vi "Axis_Initialisation.vi"(4 "Character Size":sgl=0.5, 5 "Half plane?":bool=TRUE, 6 "Axis label?":bool, 7 "Color 2":u32(colorbox)=1244928, 8 "error in (no error)":errorcluster, 9 "Radius":sgl=0.01, 10 "Length":sgl=2.0, 11 "Name":string="XYZ axis") -> (0 "error out":errorcluster, 3 "New Object Refnum":refnum<vi>)   [LabVIEW 2015]
uses:
  <vilib>/Utility/miscctls.llb/LVSceneTextAlignment.ctl
  <vilib>/picture/3D Picture Control/Object/Create Object (name).vi
  <vilib>/picture/3D Picture Control/Object/Create Object (drawable).vi
  <vilib>/picture/3D Picture Control/Object/Add Object (no reference).vi
  <vilib>/picture/3D Picture Control/NI_3D Picture Control.lvlib
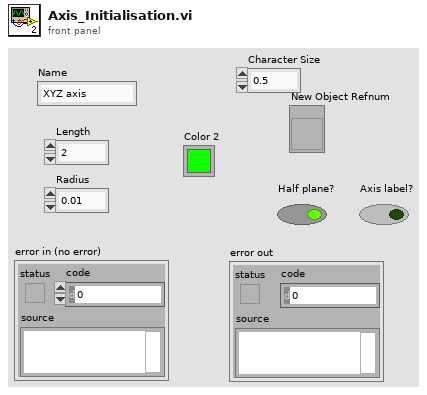
[diagram p1: front panel]
types:
  T1 = typedef "LVSceneTextAlignment.ctl" = cluster{"Horizontal Alignment":enum8{"Left", "Right", "Center"}, "Vertical Alignment":enum8{"Top", "Bottom", "Center", "Base Line", "Bottom Base Line"}}
  T2 = cluster{"Alignment":T1, "Axis Alignment":enum8{"X-Y", "Y-Z", "X-Z", "Reversed X-Y", "Reversed Y-Z", "Reversed X-Z", "Screen"}, "Vertical?":bool, "Wrap Distance":sgl}
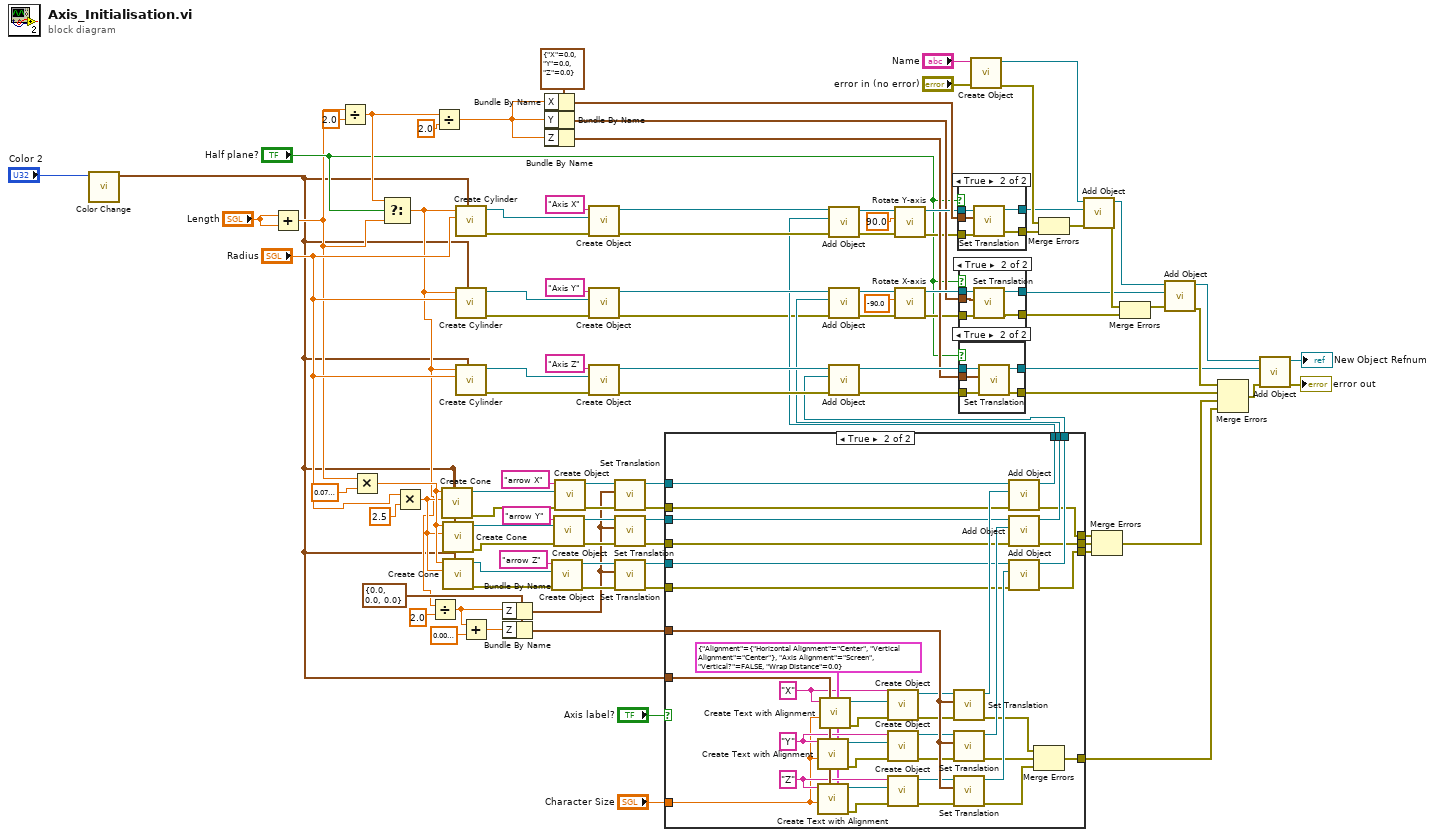
[diagram p0: block diagram]
diagram:
  w51 = cluster{"X":sgl, "Y":sgl, "Z":sgl} {"X"=0.0, "Y"=0.0, "Z"=0.0} ("Translation")
  w36 = cluster{"X":sgl, "Y":sgl, "Z":sgl} {"X"=0.0, "Y"=0.0, "Z"=0.0} ("Translation")
  n1 = call <vilib>:"Color Change.vi"("Color"="Color 2") -> ("RGBA"=w1:cluster{"R":sgl, "G":sgl, "B":sgl, "A":sgl})  [unwired: 10 in]
  n2 = Add(x="Length", y="Length") -> (x+y=w4:sgl)
  n3 = Divide(x=w4, y=sgl 2.0) -> (x/y=w72:sgl)
  n4 = Multiply(x=w4, y=sgl 0.08) -> (x*y=w14:sgl)
  n5 = Select(t=w72, s="Half plane?", f=w4) -> (s? t:f=w3:sgl)
  n6 = Multiply(x="Radius", y=sgl 2.5) -> (x*y=w13:sgl)
  n7 = Divide(x=w3, y=sgl 2.0 ("x")) -> (x/y=w15:sgl)
  n8 = Divide(x=w72, y=sgl 2.0) -> (x/y=w50:sgl)
  n9 = call <vilib>:"Create Cone.vi"("Color"=w1, "Radius"=w13, "Height"=w14) -> ("error out"=w16:errorcluster, "New Cone Refnum"=w58:refnum<vi>)  [unwired: 7 in]
  n10 = call <vilib>:"Create Cone.vi"("Color"=w1, "Radius"=w13, "Height"=w14) -> ("error out"=w9:errorcluster, "New Cone Refnum"=w11:refnum<vi>)  [unwired: 7 in]
  n11 = call <vilib>:"Create Cone.vi"("Color"=w1, "Radius"=w13, "Height"=w14) -> ("error out"=w10:errorcluster, "New Cone Refnum"=w12:refnum<vi>)  [unwired: 7 in]
  n12 = call <vilib>:"Create Cylinder.vi"("Color"=w1, "Radius"="Radius", "Height"=w3) -> ("error out"=w88:errorcluster, "New Cylinder Refnum"=w94:refnum<vi>)  [unwired: 7 in]
  n13 = call <vilib>:"Create Cylinder.vi"("Color"=w1, "Radius"="Radius", "Height"=w3) -> ("error out"=w87:errorcluster, "New Cylinder Refnum"=w96:refnum<vi>)  [unwired: 7 in]
  n14 = call <vilib>:"Create Cylinder.vi"("Color"=w1, "Radius"="Radius", "Height"=w3) -> ("error out"=w86:errorcluster, "New Cylinder Refnum"=w95:refnum<vi>)  [unwired: 7 in]
  n15 = Add(x=w15, y=sgl 0.01) -> (x+y=w27:sgl)
  n16 = Bundle By Name(cluster=w36, "Z"=w15) -> (w47:cluster{"X":sgl, "Y":sgl, "Z":sgl})
  n17 = Bundle By Name(cluster=w36, "Z"=w27) -> (w32:cluster{"X":sgl, "Y":sgl, "Z":sgl})
  n18 = Bundle By Name(cluster=w51, "X"=w50) -> (w74:cluster{"X":sgl, "Y":sgl, "Z":sgl})
  n19 = Bundle By Name(cluster=w51, "Y"=w50) -> (w52:cluster{"X":sgl, "Y":sgl, "Z":sgl})
  n20 = Bundle By Name(cluster=w51, "Z"=w50) -> (w49:cluster{"X":sgl, "Y":sgl, "Z":sgl})
  n21 = call-poly <vilib>:"Create Object.vi"("error in (no error)"=w10, "Geometry"=w12, "Name"="arrow Z") -> ("error out"=w59:errorcluster, "Scene:New Object"=w60:refnum<vi>)  [unwired: 7 in]
  n22 = call-poly <vilib>:"Create Object.vi"("error in (no error)"=w9, "Geometry"=w11, "Name"="arrow Y") -> ("error out"=w64:errorcluster, "Scene:New Object"=w63:refnum<vi>)  [unwired: 7 in]
  n23 = call-poly <vilib>:"Create Object.vi"("error in (no error)"=w16, "Geometry"=w58, "Name"="arrow X") -> ("error out"=w77:errorcluster, "Scene:New Object"=w78:refnum<vi>)  [unwired: 7 in]
  n24 = call-poly <vilib>:"Create Object.vi"("error in (no error)"=w88, "Geometry"=w94, "Name"="Axis X") -> ("error out"=w42:errorcluster, "Scene:New Object"=w67:refnum<vi>)  [unwired: 7 in]
  n25 = call-poly <vilib>:"Create Object.vi"("error in (no error)"=w87, "Geometry"=w96, "Name"="Axis Y") -> ("error out"=w19:errorcluster, "Scene:New Object"=w62:refnum<vi>)  [unwired: 7 in]
  n26 = call-poly <vilib>:"Create Object.vi"("error in (no error)"=w86, "Geometry"=w95, "Name"="Axis Z") -> ("error out"=w46:errorcluster, "Scene:New Object"=w57:refnum<vi>)  [unwired: 7 in]
  n27 = call <vilib>:"Set Translation.vi"("error in (no error)"=w77, "Translation"=w47, "Scene Object"=w78) -> ("error out"=w26:errorcluster, "Translated Object"=w38:refnum<vi>)  [unwired: 7 in]
  n28 = call <vilib>:"Set Translation.vi"("error in (no error)"=w64, "Translation"=w47, "Scene Object"=w63) -> ("error out"=w25:errorcluster, "Translated Object"=w35:refnum<vi>)  [unwired: 7 in]
  n29 = call <vilib>:"Set Translation.vi"("error in (no error)"=w59, "Translation"=w47, "Scene Object"=w60) -> ("error out"=w28:errorcluster, "Translated Object"=w33:refnum<vi>)  [unwired: 7 in]
  n30 = case shown="True" "Axis label?" {
    tunnel: w38 -> [w109 w146]
    tunnel: [w109 w145] -> w37
    tunnel: w35 -> [w108 w144]
    tunnel: [w108 w142] -> w34
    tunnel: w33 -> [w104 w141]
    tunnel: w32 -> [_ w140]
    tunnel: [w104 w138] -> w31
    tunnel: w28 -> [w106 w137]
    tunnel: w26 -> [w107 w136]
    tunnel: w25 -> [w105 w135]
    tunnel: [w107 w134] -> w24
    tunnel: [w105 w133] -> w23
    tunnel: [w106 w132] -> w22
    tunnel: [_ w131] -> w20
    tunnel: w1 -> [_ w130]
    tunnel: "Character Size" -> [_ w110]
    frame False {
    }
    frame True {
      w122 = "Z" ("text")
      w127 = "Y" ("text")
      w117 = T2 {"Alignment"={"Horizontal Alignment"=enum."Center", "Vertical Alignment"=enum."Center"}, "Axis Alignment"=enum."Screen", "Vertical?"=FALSE, "Wrap Distance"=0.0} ("Font options")
      w115 = "X" ("text")
      n31 = call <vilib>:"Create Text with Alignment.vi"("Font Options"=w117, "Color"=w130, "Character Size"=w110, "Text"=w127) -> ("error out"=w119:errorcluster, "New Text Refnum"=w126:refnum<vi>)  [unwired: 6 in]
      n32 = call <vilib>:"Create Text with Alignment.vi"("Font Options"=w117, "Color"=w130, "Character Size"=w110, "Text"=w122) -> ("error out"=w121:errorcluster, "New Text Refnum"=w123:refnum<vi>)  [unwired: 6 in]
      n33 = call <vilib>:"Create Text with Alignment.vi"("Font Options"=w117, "Color"=w130, "Character Size"=w110, "Text"=w115) -> ("error out"=w114:errorcluster, "New Text Refnum"=w129:refnum<vi>)  [unwired: 6 in]
      n34 = call-poly <vilib>:"Create Object.vi"("error in (no error)"=w114, "Geometry"=w129, "Name"=w115) -> ("error out"=w116:errorcluster, "Scene:New Object"=w128:refnum<vi>)  [unwired: 7 in]
      n35 = call-poly <vilib>:"Create Object.vi"("error in (no error)"=w119, "Geometry"=w126, "Name"=w127) -> ("error out"=w118:errorcluster, "Scene:New Object"=w125:refnum<vi>)  [unwired: 7 in]
      n36 = call-poly <vilib>:"Create Object.vi"("error in (no error)"=w121, "Geometry"=w123, "Name"=w122) -> ("error out"=w120:errorcluster, "Scene:New Object"=w124:refnum<vi>)  [unwired: 7 in]
      n37 = call <vilib>:"Set Translation.vi"("error in (no error)"=w116, "Translation"=w140, "Scene Object"=w128) -> ("error out"=w111:errorcluster, "Translated Object"=w147:refnum<vi>)  [unwired: 7 in]
      n38 = call <vilib>:"Set Translation.vi"("error in (no error)"=w118, "Translation"=w140, "Scene Object"=w125) -> ("error out"=w112:errorcluster, "Translated Object"=w143:refnum<vi>)  [unwired: 7 in]
      n39 = call <vilib>:"Set Translation.vi"("error in (no error)"=w120, "Translation"=w140, "Scene Object"=w124) -> ("error out"=w113:errorcluster, "Translated Object"=w139:refnum<vi>)  [unwired: 7 in]
      n40 = call-poly <vilib>:"Add Object.vi"("error in (no error)"=w136, "New Object In"=w147, "Scene Object In"=w146) -> ("error out"=w134:errorcluster, "Scene Object Out"=w145:refnum<vi>)  [unwired: 7 in]
      n41 = call-poly <vilib>:"Add Object.vi"("error in (no error)"=w135, "New Object In"=w143, "Scene Object In"=w144) -> ("error out"=w133:errorcluster, "Scene Object Out"=w142:refnum<vi>)  [unwired: 7 in]
      n42 = call-poly <vilib>:"Add Object.vi"("error in (no error)"=w137, "New Object In"=w139, "Scene Object In"=w141) -> ("error out"=w132:errorcluster, "Scene Object Out"=w138:refnum<vi>)  [unwired: 7 in]
      n43 = Merge Errors(w111, w112, w113) -> (w131:errorcluster)
    }
  }
  n44 = call-poly <vilib>:"Add Object.vi"("error in (no error)"=w42, "New Object In"=w37, "Scene Object In"=w67) -> ("error out"=w41:errorcluster, "Scene Object Out"=w66:refnum<vi>)  [unwired: 7 in]
  n45 = call-poly <vilib>:"Add Object.vi"("error in (no error)"=w19, "New Object In"=w34, "Scene Object In"=w62) -> ("error out"=w18:errorcluster, "Scene Object Out"=w61:refnum<vi>)  [unwired: 7 in]
  n46 = call-poly <vilib>:"Add Object.vi"("error in (no error)"=w46, "New Object In"=w31, "Scene Object In"=w57) -> ("error out"=w45:errorcluster, "Scene Object Out"=w54:refnum<vi>)  [unwired: 7 in]
  n47 = call <vilib>:"Rotate Y-axis.vi"("error in (no error)"=w41, "angle"=90.0, "Scene Object In"=w66) -> ("error out"=w40:errorcluster, "Scene Object Out"=w71:refnum<vi>)  [unwired: 7 in]
  n48 = call <vilib>:"Rotate X-axis.vi"("error in (no error)"=w18, "angle"=-90.0, "Scene Object In"=w61) -> ("error out"=w43:errorcluster, "Scene Object Out"=w56:refnum<vi>)  [unwired: 7 in]
  n49 = case shown="True" "Half plane?" {
    tunnel: w71 -> [w149 w154]
    tunnel: w74 -> [_ w153]
    tunnel: [w149 w152] -> w70
    tunnel: [w148 w151] -> w69
    tunnel: w40 -> [w148 w150]
    frame False {
    }
    frame True {
      n50 = call <vilib>:"Set Translation.vi"("error in (no error)"=w150, "Translation"=w153, "Scene Object"=w154) -> ("error out"=w151:errorcluster, "Translated Object"=w152:refnum<vi>)  [unwired: 7 in]
    }
  }
  n51 = case shown="True" "Half plane?" {
    tunnel: w56 -> [w156 w161]
    tunnel: [w156 w160] -> w55
    tunnel: [w155 w159] -> w48
    tunnel: w52 -> [_ w158]
    tunnel: w43 -> [w155 w157]
    frame False {
    }
    frame True {
      n52 = call <vilib>:"Set Translation.vi"("error in (no error)"=w157, "Translation"=w158, "Scene Object"=w161) -> ("error out"=w159:errorcluster, "Translated Object"=w160:refnum<vi>)  [unwired: 7 in]
    }
  }
  n53 = case shown="True" "Half plane?" {
    tunnel: w54 -> [w163 w168]
    tunnel: [w163 w167] -> w53
    tunnel: [w162 w166] -> w44
    tunnel: w49 -> [_ w165]
    tunnel: w45 -> [w162 w164]
    frame False {
    }
    frame True {
      n54 = call <vilib>:"Set Translation.vi"("error in (no error)"=w164, "Translation"=w165, "Scene Object"=w168) -> ("error out"=w166:errorcluster, "Translated Object"=w167:refnum<vi>)  [unwired: 7 in]
    }
  }
  n55 = call-poly <vilib>:"Create Object.vi"("error in (no error)"="error in (no error)", "Name"="Name") -> ("error out"=w85:errorcluster, "Scene:New Object"=w102:refnum<vi>)  [unwired: 8 in]
  n56 = Merge Errors(w85, w69) -> (w84:errorcluster)
  n57 = call-poly <vilib>:"Add Object.vi"("error in (no error)"=w84, "New Object In"=w70, "Scene Object In"=w102) -> ("error out"=w83:errorcluster, "Scene Object Out"=w101:refnum<vi>)  [unwired: 7 in]
  n58 = Merge Errors(w24, w23, w22) -> (w21:errorcluster)
  n59 = Merge Errors(w83, w48) -> (w82:errorcluster)
  n60 = call-poly <vilib>:"Add Object.vi"("error in (no error)"=w82, "New Object In"=w55, "Scene Object In"=w101) -> ("error out"=w81:errorcluster, "Scene Object Out"=w100:refnum<vi>)  [unwired: 7 in]
  n61 = Merge Errors(w81, w44, w21, w20) -> (w80:errorcluster)
  n62 = call-poly <vilib>:"Add Object.vi"("error in (no error)"=w80, "New Object In"=w53, "Scene Object In"=w100) -> ("error out"=→"error out":errorcluster, "Scene Object Out"=→"New Object Refnum":refnum<vi>)  [unwired: 7 in]
